vi "Save data file to network drive v4.vi"(8 "Input Cluster":T1, 11 "panel id":string) -> (0 "network file save error":errorcluster, 3 "file save path":string)   [LabVIEW 2013]
uses:
  program files/Global 1.vi
panel:
  out "status":string
  out "C drive root path":string
  out "network file dir path":path
  out "network dir":string
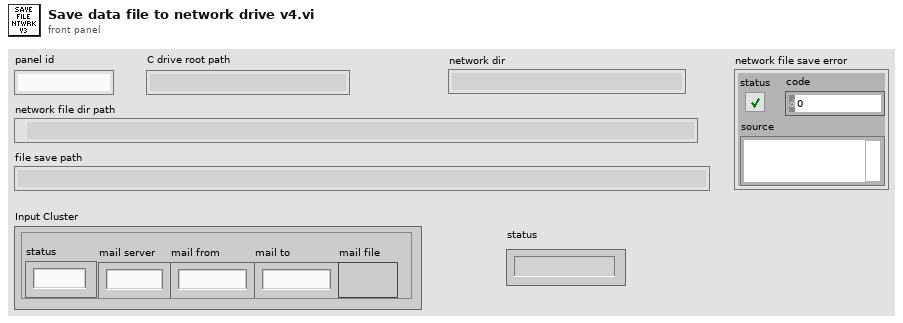
[diagram p1: front panel]
types:
  T1 = cluster{"status":string, "mail server":string, "mail from":string, "mail to":string, "mail file":bool}
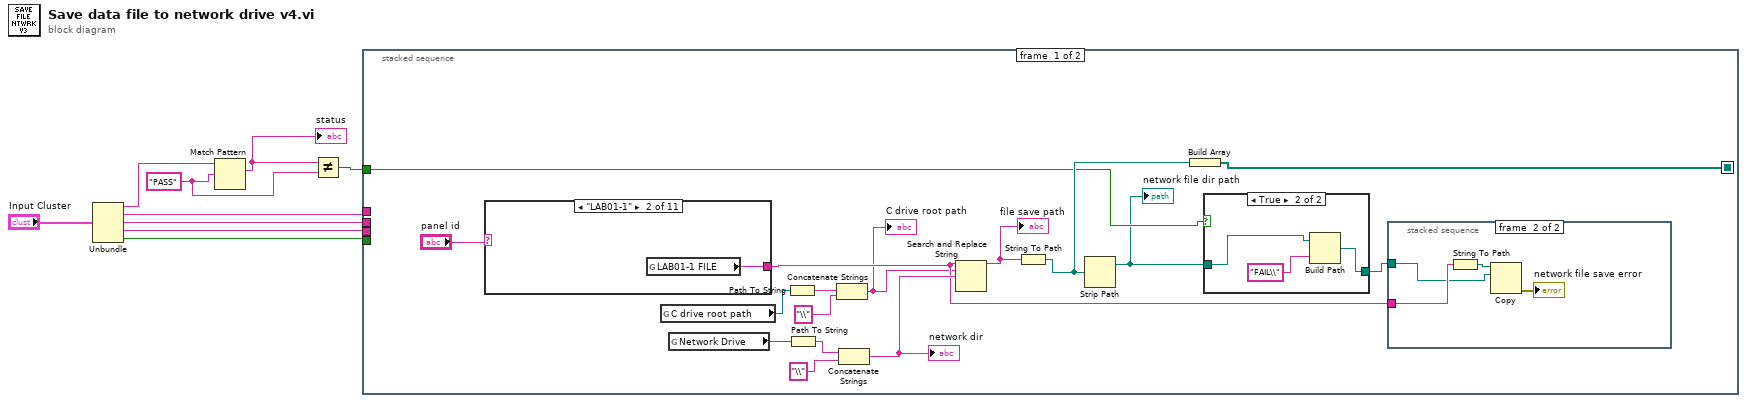
[diagram p0: block diagram]
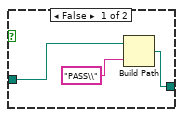
[diagram p2: hidden frame]
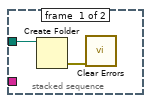
[diagram p3: hidden frame]
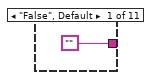
[diagram p4: hidden frame]
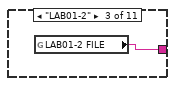
[diagram p5: hidden frame]
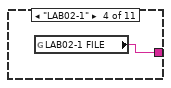
[diagram p6: hidden frame]
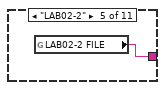
[diagram p7: hidden frame]
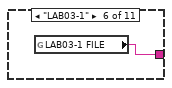
[diagram p8: hidden frame]
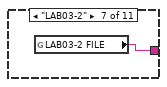
[diagram p9: hidden frame]
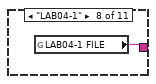
[diagram p10: hidden frame]
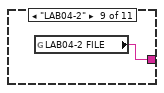
[diagram p11: hidden frame]
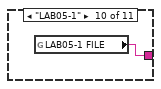
[diagram p12: hidden frame]
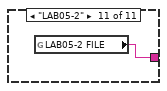
[diagram p13: hidden frame]
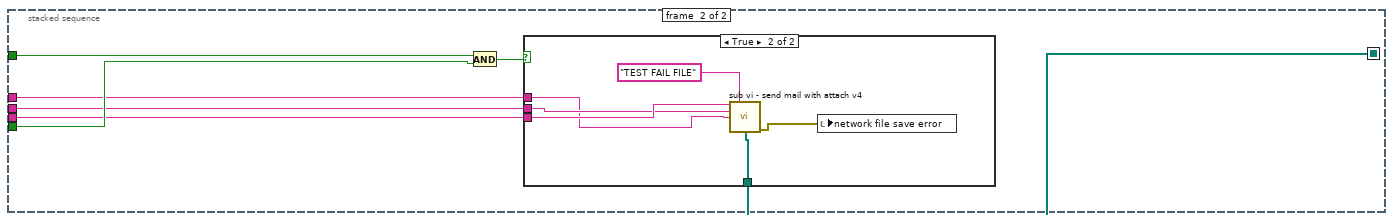
[diagram p14: hidden frame]
diagram:
  w9 = "PASS"
  n1 = Unbundle("Input Cluster") -> ("status"=w7:string, "mail server"=w1:string, "mail from"=w2:string, "mail to"=w3:string, "mail file"=w4:bool)
  n2 = Match Pattern(string=w7, regular expression=w9) -> (match substring=w8:string)  [unwired: 1 in, 3 out]
  "status" <- w8
  n3 = Not Equal?(x=w8, y=w9) -> (x != y?=w5:bool)
  n4 = stacked-sequence {
    seq-local: [w13 _] -> [_ w54]
    tunnel: w5 -> [w12 w53]
    tunnel: w4 -> [_ w52]
    tunnel: w3 -> [_ w51]
    tunnel: w2 -> [_ w50]
    tunnel: w1 -> [_ w49]
    frame #0 {
      n5 = case shown="\"LAB01-1\"" "panel id" {
        tunnel: ["" w39 w40 w41 w42 w43 w44 w45 w46 w47 w48] -> w19
        frame "False", Default {
        }
        frame "LAB01-1" {
          n6 = global read "Global 1.vi" "LAB01-1 FILE"() -> (w39:string)
        }
        frame "LAB01-2" {
          n7 = global read "Global 1.vi" "LAB01-2 FILE"() -> (w40:string)
        }
        frame "LAB02-1" {
          n8 = global read "Global 1.vi" "LAB02-1 FILE"() -> (w41:string)
        }
        frame "LAB02-2" {
          n9 = global read "Global 1.vi" "LAB02-2 FILE"() -> (w42:string)
        }
        frame "LAB03-1" {
          n10 = global read "Global 1.vi" "LAB03-1 FILE"() -> (w43:string)
        }
        frame "LAB03-2" {
          n11 = global read "Global 1.vi" "LAB03-2 FILE"() -> (w44:string)
        }
        frame "LAB04-1" {
          n12 = global read "Global 1.vi" "LAB04-1 FILE"() -> (w45:string)
        }
        frame "LAB04-2" {
          n13 = global read "Global 1.vi" "LAB04-2 FILE"() -> (w46:string)
        }
        frame "LAB05-1" {
          n14 = global read "Global 1.vi" "LAB05-1 FILE"() -> (w47:string)
        }
        frame "LAB05-2" {
          n15 = global read "Global 1.vi" "LAB05-2 FILE"() -> (w48:string)
        }
      }
      n16 = global read "Global 1.vi" "C drive root path"() -> (w16:path)
      n17 = global read "Global 1.vi" "Network Drive"() -> (w24:path)
      n18 = Path To String(path=w16) -> (string=w17:string)
      n19 = Path To String(path=w24) -> (string=w23:string)
      n20 = Concatenate Strings(w17, "\\") -> (w15:string)
      "C drive root path" <- w15
      n21 = Concatenate Strings(w23, "\\") -> (w21:string)
      "network dir" <- w21
      n22 = Search and Replace String(input string=w19, search string=w15, replace string=w21) -> (result string=w20:string)  [unwired: 5 in, 3 out]
      "file save path" <- w20
      n23 = String To Path(string=w20) -> (path=w14:path)
      n24 = Strip Path(path=w14) -> (stripped path=w10:path)  [unwired: 1 out]
      "network file dir path" <- w10
      n25 = Build Array(w14) -> (w13:path[])
      n26 = case shown="True" w12 {
        tunnel: [w26 w31] -> w11
        tunnel: w10 -> [w27 w29]
        frame False {
          n27 = Build Path(base path=w27, name or relative path="PASS\\") -> (appended path=w26:path)
        }
        frame True {
          n28 = Build Path(base path=w29, name or relative path="FAIL\\") -> (appended path=w31:path)
        }
      }
      n29 = stacked-sequence {
        tunnel: w11 -> [w33 w34]
        tunnel: w19 -> [_ w35]
        frame #0 {
          n30 = Create Folder(path (use dialog)=w33) -> (error out=w32:errorcluster)  [unwired: 2 in, 2 out]
          n31 = call <vilib>:"Clear Errors.vi"("error in (no error)"=w32) -> ()  [unwired: 6 in, 1 out]
        }
        frame #1 {
          n32 = String To Path(string=w35) -> (path=w36:path)
          n33 = Copy(10:w34, 11:w36) -> (0:→"network file save error":errorcluster)  [unwired: 3 in, 2 out]
        }
      }
    }
    frame #1 {
      n34 = And(x=w53, y=w52) -> (x .and. y?=w55:bool)
      n35 = case shown="True" w55 {
        tunnel: w54 -> [_ w60]
        tunnel: w51 -> [_ w58]
        tunnel: w50 -> [_ w57]
        tunnel: w49 -> [_ w56]
        frame False {
        }
        frame True {
          n36 = call "sub vi - send mail with attach v4.vi"("TO:"=w58, "subject"="TEST FAIL FILE", "from"=w57, "out going server"=w56, "Attachements"=w60) -> ("error out"=w61:errorcluster)  [unwired: 10 in]
          n37 = local write "network file save error"(w61) -> ()
        }
      }
    }
  }
